vi "2D arrays.vi"() -> ()   [LabVIEW 2024]
panel:
  out "Array 6":dbl[][](array[numeric])
  out "Array":dbl[](array[numeric])
  out "Array 5":bool[](array[boolean])
  in  "Array 4":bool[](array[boolean])
  out "Array 3":dbl[](array[numeric])
  in  "Array 2":dbl[](array[numeric])
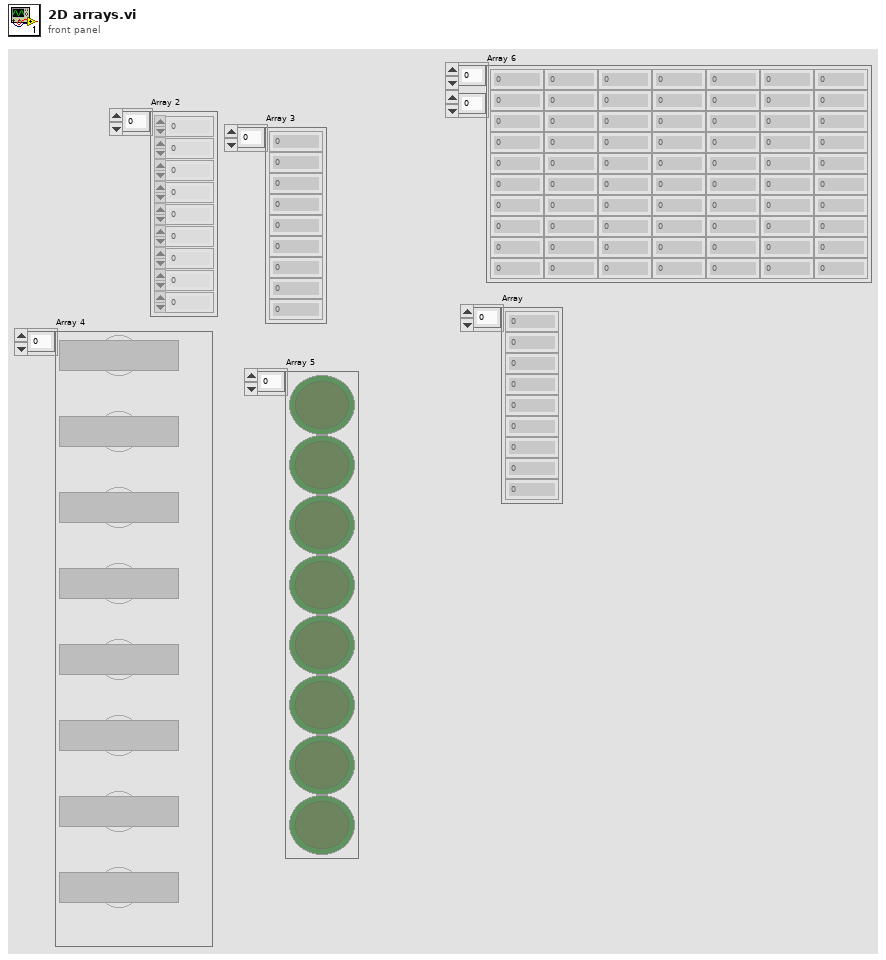
[diagram p1: front panel]
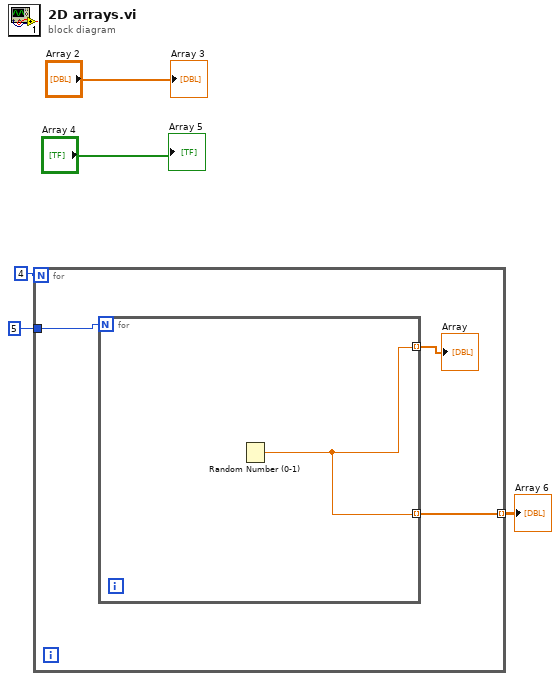
[diagram p0: block diagram]
diagram:
  n1 = for {
    N: 4 -> [_]
    tunnel: [w8] -> w1 mode=indexing
    tunnel: 5 -> [w7]
    n2 = for {
      N: w7 -> [_]
      tunnel: [w9] -> w6 mode=indexing
      tunnel: [w9] -> w8 mode=indexing
      n3 = Random Number (0-1)() -> (number: 0 to 1=w9:dbl)
    }
    "Array" <- w6
  }
  "Array 6" <- w1
  "Array 5" <- "Array 4"
  "Array 3" <- "Array 2"
